vi "Ventile manuell schalten Crio.vi"(8 "error in (no error)":errorcluster caption="Fehler (Eingang, kein Fehler)", 11 "DO 0-31":T1) -> (0 "error out":errorcluster caption="Fehler (Ausgang)", 3 "DO 0-31":T1)   [LabVIEW 2020, in "Allgemein.lvlib"]
uses:
  Allgemein.lvlib
  Verwaltung/Digital Ausgaenge 0-31.ctl
  Verwaltung/Verwaltung - cRIO.lvlib
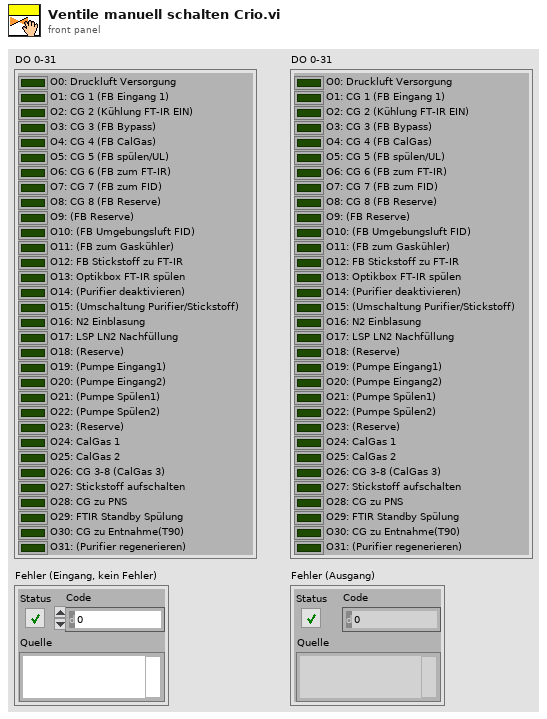
[diagram p1: front panel]
types:
  T1 = typedef "Verwaltung - cRIO.lvlib/Digital Ausgaenge 0-31.ctl" = cluster{"O0: Druckluft Versorgung":bool, "O1: CG 1 (FB Eingang 1)":bool, "O2: CG 2 (Kühlung FT-IR EIN)":bool, "O3: CG 3 (FB Bypass)":bool, "O4: CG 4 (FB CalGas)":bool, "O5: CG 5 (FB spülen/UL)":bool, "O6: CG 6 (FB zum FT-IR)":bool, "O7: CG 7 (FB zum FID)":bool, "O8: CG 8 (FB Reserve)":bool, "O9: (FB Reserve)":bool, "O10: (FB Umgebungsluft FID)":bool, "O11: (FB zum Gaskühler)":bool, "O12: FB Stickstoff zu FT-IR":bool, "O13: Optikbox FT-IR spülen":bool, "O14: (Purifier deaktivieren)":bool, "O15: (Umschaltung Purifier/Stickstoff)":bool, "O16: N2 Einblasung":bool, "O17: LSP LN2 Nachfüllung":bool, "O18: (Reserve)":bool, "O19: (Pumpe Eingang1)":bool, "O20: (Pumpe Eingang2)":bool, "O21: (Pumpe Spülen1)":bool, "O22: (Pumpe Spülen2)":bool, "O23: (Reserve)":bool, "O24: CalGas 1":bool, "O25: CalGas 2":bool, "O26: CG 3-8 (CalGas 3)":bool, "O27: Stickstoff aufschalten":bool, "O28: CG zu PNS":bool, "O29: FTIR Standby Spülung":bool, "O30: CG zu Entnahme(T90)":bool, "O31: (Purifier regenerieren)":bool}
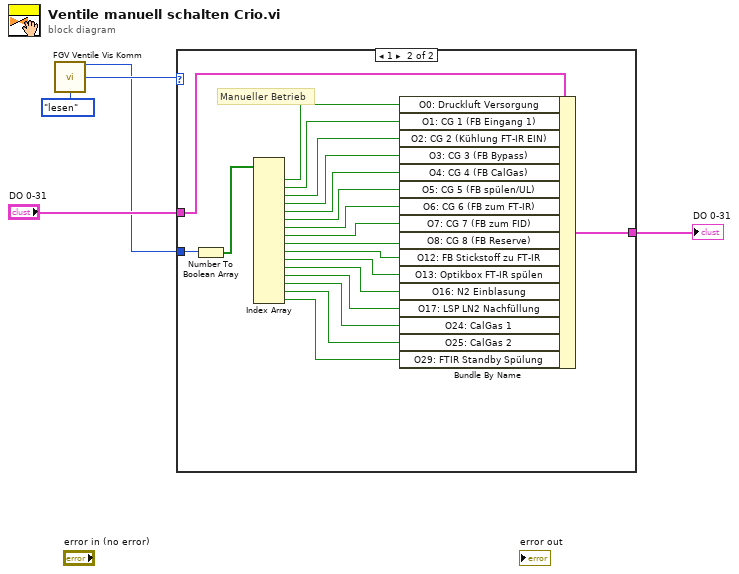
[diagram p0: block diagram]
diagram:
  n1 = call "FGV Ventile Vis Komm.vi"("Aktion"=enum16{"lesen", "schreiben"}."lesen") -> ("Ventile schalten"=w2:u32, "Betrieb"=w3:u16)  [unwired: 12 in, 1 out]
  n2 = case shown="1" w3 {
    tunnel: "DO 0-31" -> [w6 w26]
    tunnel: w2 -> [_ w24]
    tunnel: [w6 w25] -> w1
    frame 0, Default {
      # "Normaler Betrieb"
    }
    frame 1 {
      # "Manueller Betrieb"
      n3 = Number To Boolean Array(number=w24) -> (Boolean array=w23:bool[])
      n4 = Index Array(array=w23) -> (element #1=w22:bool, element #2=w21:bool, element #3=w20:bool, element #4=w19:bool, element #5=w18:bool, element #6=w17:bool, element #7=w16:bool, element #8=w15:bool, element #9=w14:bool, element #10=w13:bool, element #11=w12:bool, element #12=w11:bool, element #13=w10:bool, element #14=w9:bool, element #15=w8:bool, element #16=w7:bool)  [unwired: 16 in]
      n5 = Bundle By Name(cluster=w26, "O0: Druckluft Versorgung"=w22, "O1: CG 1 (FB Eingang 1)"=w21, "O2: CG 2 (Kühlung FT-IR EIN)"=w20, "O3: CG 3 (FB Bypass)"=w19, "O4: CG 4 (FB CalGas)"=w18, "O5: CG 5 (FB spülen/UL)"=w17, "O6: CG 6 (FB zum FT-IR)"=w16, "O7: CG 7 (FB zum FID)"=w15, "O8: CG 8 (FB Reserve)"=w14, "O12: FB Stickstoff zu FT-IR"=w13, "O13: Optikbox FT-IR spülen"=w12, "O16: N2 Einblasung"=w11, "O17: LSP LN2 Nachfüllung"=w10, "O24: CalGas 1"=w9, "O25: CalGas 2"=w8, "O29: FTIR Standby Spülung"=w7) -> (w25:T1)
    }
  }
  "DO 0-31" <- w1
